vi "LVClass_HasoField dtor.vi"(0 "HasoField in":refnum<class "HasoField.lvclass">, 11 "error in (no error)":errorcluster) -> (4 "HasoField out":refnum<class "HasoField.lvclass">, 15 "error out":errorcluster)   [LabVIEW 2020, in "HasoField.lvclass"]
doc: "HasoField destructor.\n\n--------------------------------------------------------------------------------\n\n<B>HasoFieldIn </B> : HasoField object.\n<B>HasoFieldOut </B> : HasoField object.\n<B>ErrorIn </B> : Error\n<B>ErrorOut </B> : Error\n\n--------------------------------------------------------------------------------"
uses:
  HasoField.lvclass
  HasoField.lvclass/HasoField.ctl
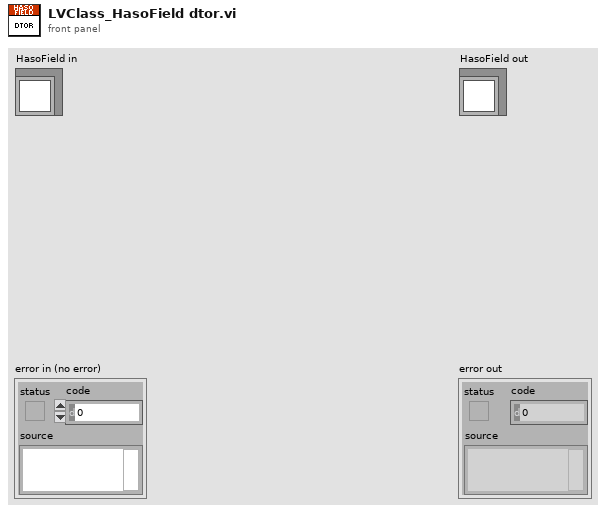
[diagram p1: front panel]
types:
  T1 = typedef "Handle creation.ctl" = enum16{"By ctor", "By write function"}
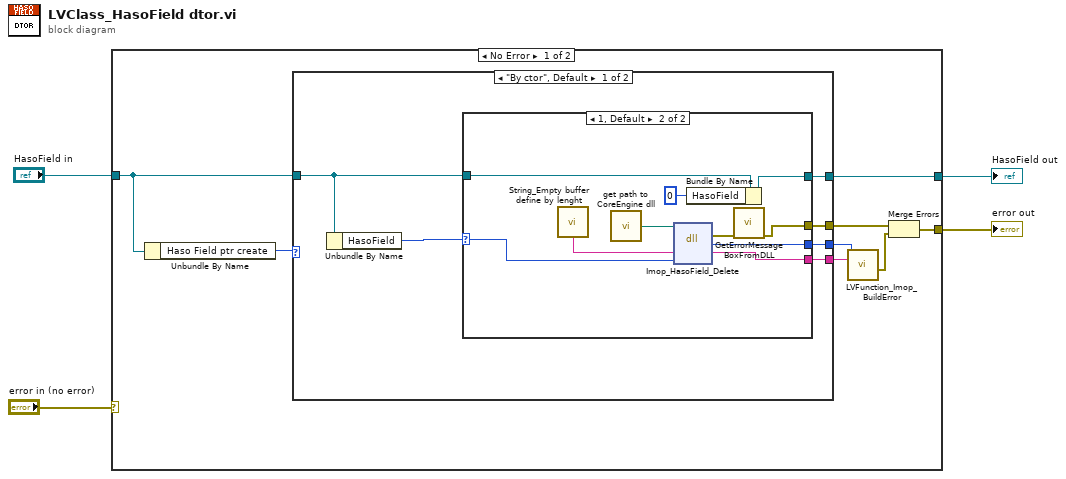
[diagram p0: block diagram]
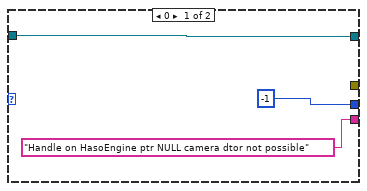
[diagram p2: hidden frame]
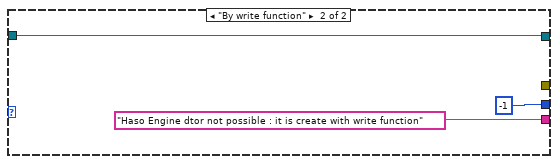
[diagram p3: hidden frame]
diagram:
  n1 = case shown="No Error" "error in (no error)" {
    selector: "error in (no error)" -> [_ w35]
    tunnel: "HasoField in" -> [w5 w36]
    tunnel: [w10 w36] -> w4
    tunnel: [w6 w35] -> w2
    frame No Error {
      n2 = Unbundle By Name(w5) -> ("Haso Field ptr create"=w9:T1)
      n3 = case shown="\"By ctor\", Default" w9 {
        tunnel: [w18 "Haso Engine dtor not possible : it is create with write function" ("message")] -> w12
        tunnel: [w17 -1] -> w11
        tunnel: w5 -> [w15 w32]
        tunnel: [w16 w32] -> w10
        tunnel: [w13 _] -> w8
        frame "By ctor", Default {
          n4 = Unbundle By Name(w15) -> ("HasoField"=w14:i32)
          n5 = case shown="1, Default" w14 {
            selector: w14 -> [_ w28]
            tunnel: ["Handle on HasoEngine ptr NULL camera dtor not possible" ("message") w30] -> w18
            tunnel: [-1 w29] -> w17
            tunnel: w15 -> [w19 w24]
            tunnel: [w19 w23] -> w16
            tunnel: [_ w22] -> w13
            frame 0 {
            }
            frame 1, Default {
              n6 = call "String_Empty buffer define by lenght.vi"() -> ("Empty buffer"=w31:string)  [unwired: 1 in]
              n7 = call "get path to CoreEngine dll.vi"() -> ("path to c_interface_vc100.dll"=w27:path)  [unwired: 12 in, 3 out]
              n8 = dll-call lib="D:/soft/HASO_v3/SVN_trunk/ImOpCoreEngine4_LV2011/DLLs/c_interface_vc100.dll" fn="Imop_HasoField_Delete"(path in=w27, "message"=w31, "objet"=w28) -> (error out=w26:errorcluster, "return type"=w29:i32, "message"=w30:string)  [unwired: 3 in, 1 out]
              n9 = Bundle By Name(cluster=w24, "HasoField"=u32 0 ("HasoEgine")) -> (w23:refnum<class "HasoField.lvclass">)
              n10 = call "GetErrorMessageBoxFromDLL.vi"("error IN"=w26) -> ("error OUT"=w22:errorcluster)  [unwired: 10 in]
            }
          }
        }
        frame "By write function" {
        }
      }
      n11 = call "LVFunction_Imop_BuildError.vi"("code"=w11, "String to Prepend to source (\"\")"=w12) -> ("error out"=w7:errorcluster)  [unwired: 13 in]
      n12 = Merge Errors(w8, w7) -> (w6:errorcluster)
    }
    frame Error {
    }
  }
  "error out" <- w2
  "HasoField out" <- w4
